vi "Abadines_Server5.vi"() -> ()   [LabVIEW 2013]
uses:
  <vilib>/NXT/Block Support/NXT_InputPort.ctl
  <vilib>/NXT/Block Support/NXT_MessageMailbox.ctl
  <vilib>/NXT/Block Support/NXT_OutputPort.ctl
  <vilib>/NXT/Subs/MotorOutput.ctl
  <vilib>/NXT/Dual Mode Library/BT/BlueTooth_Write_Num.vi
  <vilib>/NXT/NXTIO Xnodes/NXTIONodeSubVIs/NXTStopMotors.vi
  <vilib>/NXT/Dual Mode Library/Display/drawNumber.vi
  <vilib>/NXT/NXTIO Xnodes/AddressXNode/NXTIOAddress.xnode
  <vilib>/NXT/NXTIO Xnodes/NXTIOXNode/NXTIO.xnode
  <vilib>/NXT/Subs/LVHSConnector.ctl
  <vilib>/NXT/LegoClasses/BrickReference/BrickReference.lvclass
panel:
  out "Blue Line":i16
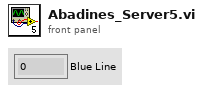
[diagram p1: front panel]
types:
  T1 = typedef "NXT_OutputPort.ctl" = u8
  T2 = typedef "NXT_InputPort.ctl" = u32
  T3 = typedef "LVHSConnector.ctl" = refnum<class "BrickReference.lvclass">
  T4 = typedef "NXT_MessageMailbox.ctl" = u8
  T5 = typedef "MotorOutput.ctl" = u8
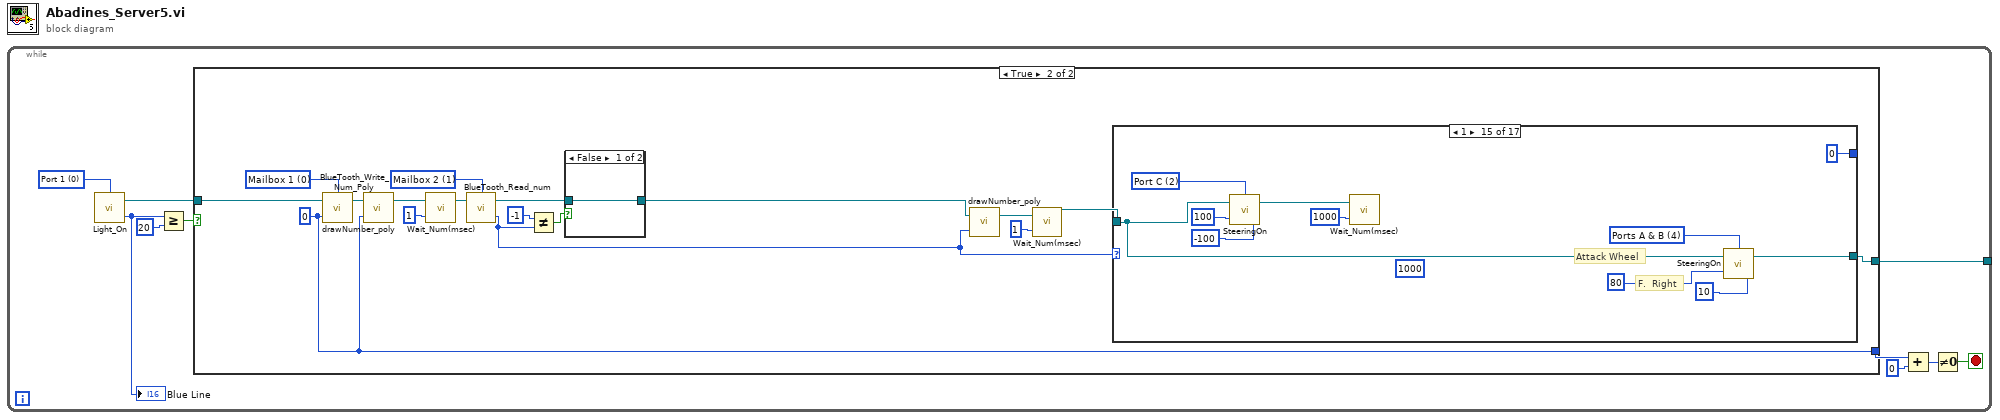
[diagram p0: block diagram]
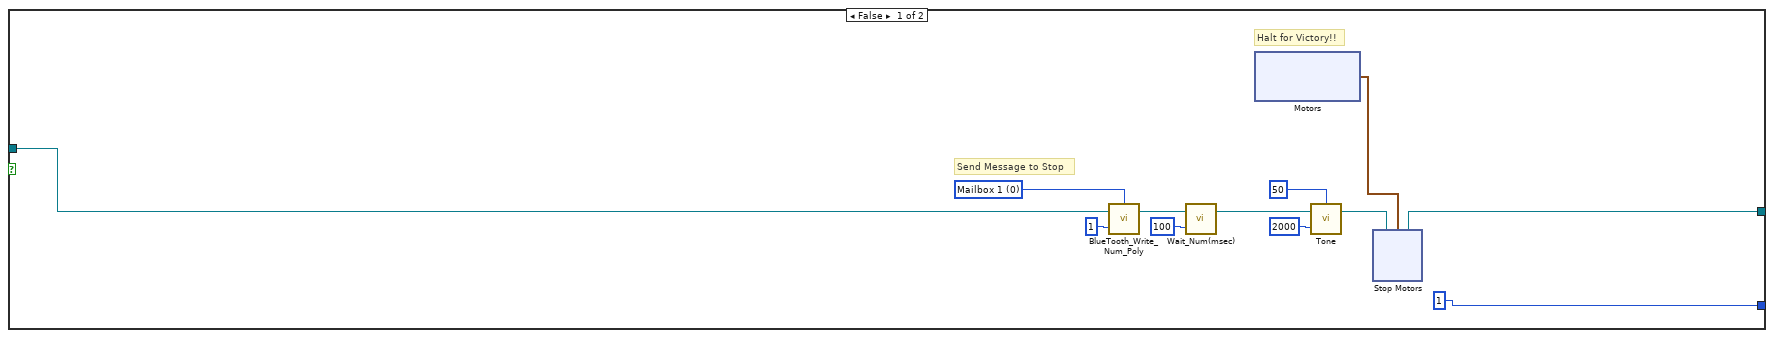
[diagram p2: hidden frame]
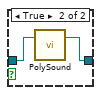
[diagram p3: hidden frame]
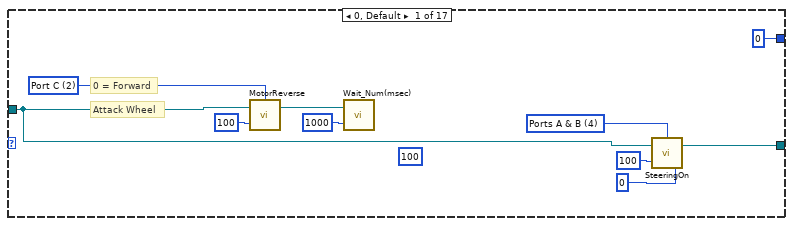
[diagram p4: hidden frame]
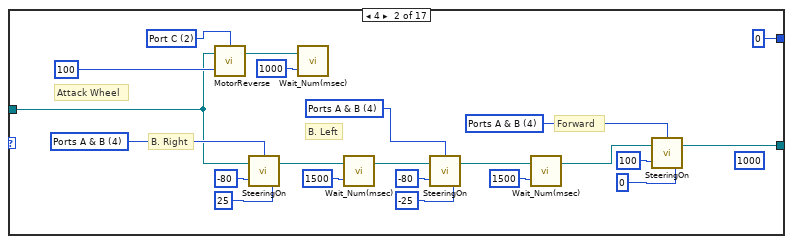
[diagram p5: hidden frame]
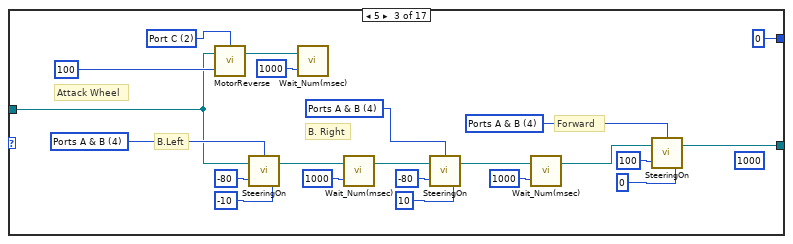
[diagram p6: hidden frame]
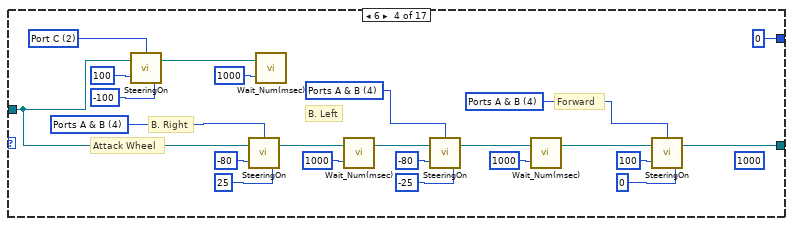
[diagram p7: hidden frame]
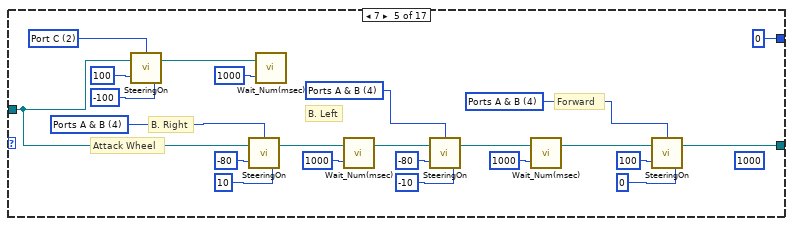
[diagram p8: hidden frame]
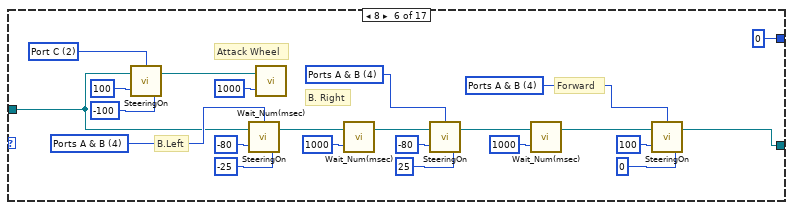
[diagram p9: hidden frame]
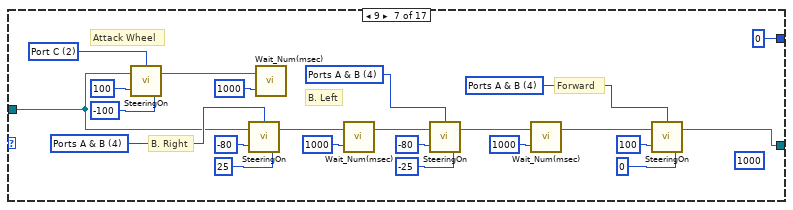
[diagram p10: hidden frame]
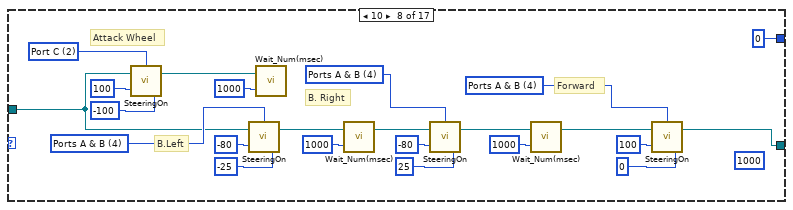
[diagram p11: hidden frame]
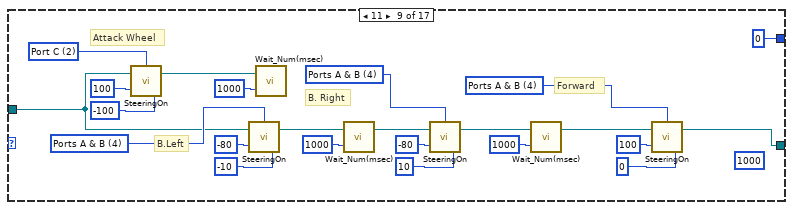
[diagram p12: hidden frame]
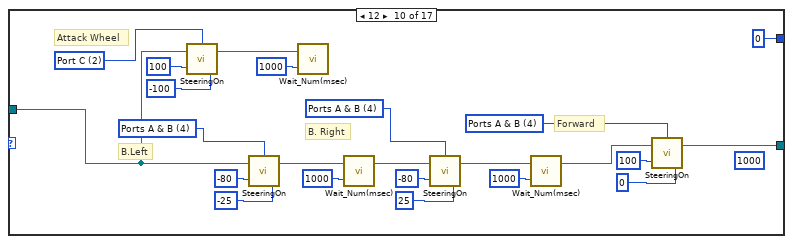
[diagram p13: hidden frame]
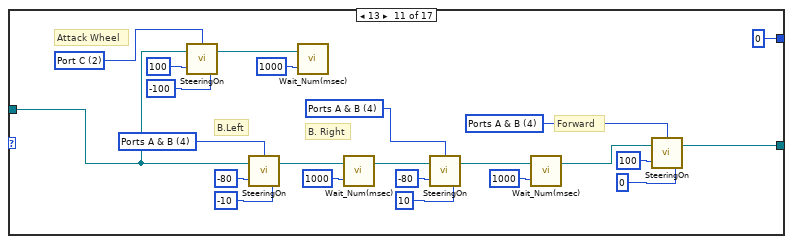
[diagram p14: hidden frame]
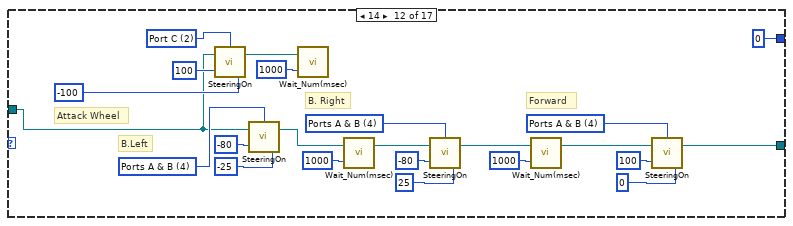
[diagram p15: hidden frame]
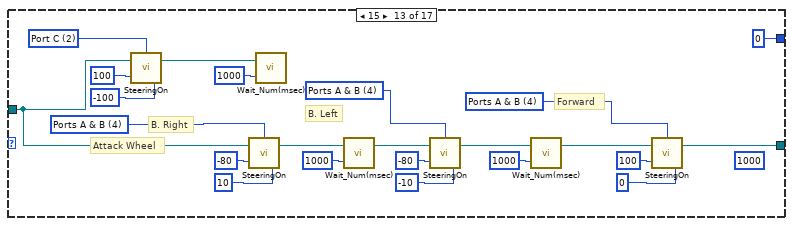
[diagram p16: hidden frame]
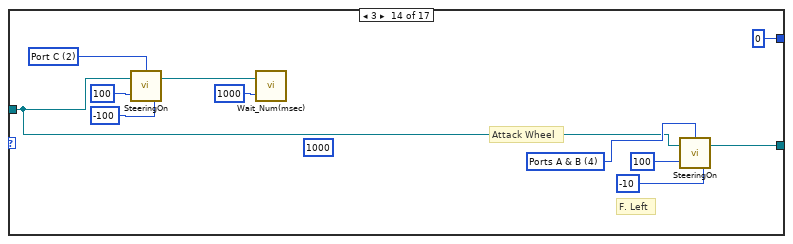
[diagram p17: hidden frame]
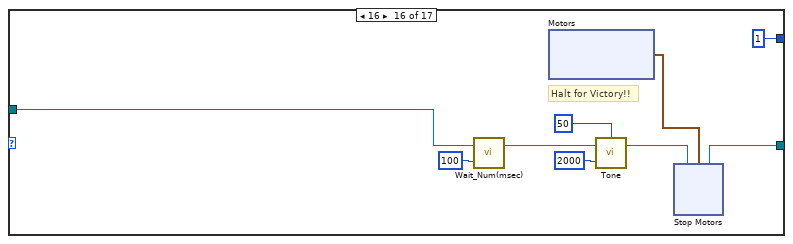
[diagram p18: hidden frame]
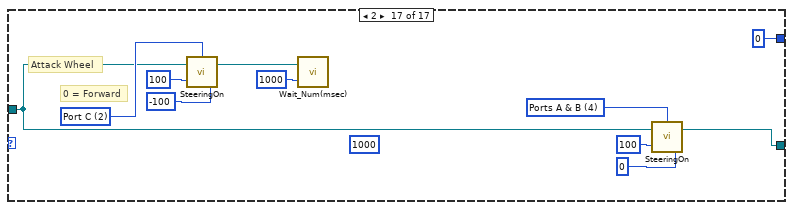
[diagram p19: hidden frame]
diagram:
  n1 = while {
    tunnel: [w6] -> _
    stop <- w2 stop-if-true
    w10 = T2 0 items=["Port 1", "Port 2", "Port 3", "Port 4"] ("Port (Port 3)")
    n2 = call <vilib>:"Light_On.vi"("Port (Port 3)"=w10) -> ("Scaled Value"=w9:i16, "NXT/EV3"=w1:T3)  [unwired: 2 in]
    "Blue Line" <- w9
    n3 = Greater Or Equal?(x=w9, y=i16 20) -> (x >= y?=w7:bool)
    n4 = case shown="True" w7 {
      tunnel: w1 -> [w20 w38]
      tunnel: [w14 w36] -> w6
      tunnel: [1 w35] -> w5
      frame False {
        w21 = T4 0 items=["Mailbox 1", "Mailbox 2", "Mailbox 3", "Mailbox 4", "Mailbox 5", "Mailbox 6", "Mailbox 7", "Mailbox 8", "Mailbox 9", "Mailbox 10"] ("Mailbox")
        # "Halt for Victory!!"
        # "Send Message to Stop"
        n5 = call-poly <vilib>:"BlueTooth_Write_Num_Poly.vi"("Message"=1, "NXT/EV3"=w20, "Mailbox"=w21) -> ("NXT/EV3"=w16:T3)  [unwired: 1 in]
        n6 = call <vilib>:"Wait_Num(msec).vi"("Time (100 msec)"=u32 100, "NXT/EV3"=w16) -> ("NXT/EV3"=w17:T3)  [unwired: 2 in]
        n7 = xnode "Motors"() -> ("Motor"=w13:cluster{"Port":T1, "Port":T1})
        n8 = call <vilib>:"Tone.vi"("Duration (500 ms)"=u16 2000, "NXT/EV3"=w17, "Tone (440 Hz)"=u16 50) -> ("NXT/EV3"=w15:T3)  [unwired: 1 in]
        n9 = xnode "Stop Motors"("Motors"=w13, "NXT/EV3"=w15) -> ("NXT/EV3"=w14:T3)
      }
      frame True {
        w45 = T4 1 items=["Mailbox 1", "Mailbox 2", "Mailbox 3", "Mailbox 4", "Mailbox 5", "Mailbox 6", "Mailbox 7", "Mailbox 8", "Mailbox 9", "Mailbox 10"] ("Mailbox")
        w35 = 0 ("Message")
        w39 = T4 0 items=["Mailbox 1", "Mailbox 2", "Mailbox 3", "Mailbox 4", "Mailbox 5", "Mailbox 6", "Mailbox 7", "Mailbox 8", "Mailbox 9", "Mailbox 10"] ("Mailbox")
        n10 = call-poly <vilib>:"BlueTooth_Write_Num_Poly.vi"("Message"=w35, "NXT/EV3"=w38, "Mailbox"=w39) -> ("NXT/EV3"=w32:T3)  [unwired: 1 in]
        n11 = call-poly <vilib>:"drawNumber_poly.vi"("number"=w35, "NXT/EV3"=w32) -> ("NXT/EV3"=w40:T3)  [unwired: 2 in]
        n12 = call <vilib>:"Wait_Num(msec).vi"("Time (100 msec)"=u32 1, "NXT/EV3"=w40) -> ("NXT/EV3"=w41:T3)  [unwired: 2 in]
        n13 = call <vilib>:"BlueTooth_Read_num.vi"("NXT/EV3"=w41, "Mailbox"=w45) -> ("Message"=w31:i32, "NXT/EV3"=w30:T3)  [unwired: 1 in]
        n14 = Not Equal?(x=-1, y=w31) -> (x != y?=w33:bool)
        n15 = case shown="False" w33 {
          tunnel: [w46 w48] -> w29
          tunnel: w30 -> [w46 w47]
          frame False {
          }
          frame True {
            n16 = call-poly <vilib>:"PolySound.vi"("NXT/EV3"=w47) -> ("NXT/EV3"=w48:T3)  [unwired: 3 in]
          }
        }
        n17 = call-poly <vilib>:"drawNumber_poly.vi"("number"=w31, "NXT/EV3"=w29) -> ("NXT/EV3"=w44:T3)  [unwired: 2 in]
        n18 = call <vilib>:"Wait_Num(msec).vi"("Time (100 msec)"=u32 1, "NXT/EV3"=w44) -> ("NXT/EV3"=w37:T3)  [unwired: 2 in]
        n19 = case shown="1" w31 {
          tunnel: [w56 w74 w87 w110 w133 w165 w179 w202 w225 w249 w271 w294 w318 w341 w352 w361 w378] -> w36
          tunnel: w37 -> [w49 w59 w81 w103 w126 w149 w172 w195 w218 w242 w265 w287 w310 w333 w344 w357 w371]
          tunnel: [0 ("Steering (100)") 0 ("Steering (100)") 0 ("Steering (100)") 0 ("Steering (100)") 0 ("Steering (100)") 0 ("Steering (100)") 0 ("Steering (100)") 0 ("Steering (100)") 0 ("Steering (100)") 0 ("Steering (100)") 0 ("Steering (100)") 0 ("Steering (100)") 0 ("Steering (100)") 0 ("Steering (100)") 0 ("Steering (100)") 1 ("Steering (100)") 0 ("Steering (100)")] -> _
          frame 0, Default {
            (unwired) u16 100 ("Duration (500 ms)")
            w54 = T5 2 items=["Port A"=0, "Port B"=1, "Port C"=2, "Ports A & B"=4, "Ports A & C"=5, "Ports B & C"=6, "All Ports"=3] ("Output Ports (A & B)")
            w55 = T5 4 items=["Port A"=0, "Port B"=1, "Port C"=2, "Ports A & B"=4, "Ports A & C"=5, "Ports B & C"=6, "All Ports"=3] ("Output Ports (A & B) 5")
            # "Attack Wheel"
            # "0 = Forward"
            n20 = call <vilib>:"MotorReverse.vi"("Power (75)"=100, "NXT/EV3"=w49, "Output Port (All Ports)"=w54) -> ("NXT/EV3"=w52:T3)  [unwired: 1 in]
            n21 = call <vilib>:"Wait_Num(msec).vi"("Time (100 msec)"=u32 1000, "NXT/EV3"=w52) -> ()  [unwired: 2 in, 1 out]
            n22 = call <vilib>:"SteeringOn.vi"("Power (75)"=100, "Steering (100)"=0, "NXT/EV3"=w49, "Output Ports (A & B)"=w55) -> ("NXT/EV3"=w56:T3)
          }
          frame 4 {
            (unwired) u16 1000 ("Duration (500 ms)")
            w64 = T5 2 items=["Port A"=0, "Port B"=1, "Port C"=2, "Ports A & B"=4, "Ports A & C"=5, "Ports B & C"=6, "All Ports"=3] ("Output Ports (A & B)")
            w71 = T5 4 items=["Port A"=0, "Port B"=1, "Port C"=2, "Ports A & B"=4, "Ports A & C"=5, "Ports B & C"=6, "All Ports"=3] ("Output Ports (A & B) 15")
            w72 = T5 4 items=["Port A"=0, "Port B"=1, "Port C"=2, "Ports A & B"=4, "Ports A & C"=5, "Ports B & C"=6, "All Ports"=3] ("Output Port (All Ports) 6")
            w73 = T5 4 items=["Port A"=0, "Port B"=1, "Port C"=2, "Ports A & B"=4, "Ports A & C"=5, "Ports B & C"=6, "All Ports"=3] ("Output Ports (A & B) 16")
            # "Attack Wheel"
            # "Forward"
            # "B. Left"
            # "B. Right"
            n23 = call <vilib>:"MotorReverse.vi"("Power (75)"=100, "NXT/EV3"=w59, "Output Port (All Ports)"=w64) -> ("NXT/EV3"=w62:T3)  [unwired: 1 in]
            n24 = call <vilib>:"SteeringOn.vi"("Power (75)"=-80, "Steering (100)"=25, "NXT/EV3"=w59, "Output Ports (A & B)"=w73) -> ("NXT/EV3"=w70:T3)
            n25 = call <vilib>:"Wait_Num(msec).vi"("Time (100 msec)"=u32 1000, "NXT/EV3"=w62) -> ()  [unwired: 2 in, 1 out]
            n26 = call <vilib>:"Wait_Num(msec).vi"("Time (100 msec)"=u32 1500, "NXT/EV3"=w70) -> ("NXT/EV3"=w69:T3)  [unwired: 2 in]
            n27 = call <vilib>:"SteeringOn.vi"("Power (75)"=-80, "Steering (100)"=-25, "NXT/EV3"=w69, "Output Ports (A & B)"=w72) -> ("NXT/EV3"=w68:T3)
            n28 = call <vilib>:"Wait_Num(msec).vi"("Time (100 msec)"=u32 1500, "NXT/EV3"=w68) -> ("NXT/EV3"=w67:T3)  [unwired: 2 in]
            n29 = call <vilib>:"SteeringOn.vi"("Power (75)"=100, "Steering (100)"=0, "NXT/EV3"=w67, "Output Ports (A & B)"=w71) -> ("NXT/EV3"=w74:T3)
          }
          frame 5 {
            (unwired) u16 1000 ("Duration (500 ms)")
            w86 = T5 2 items=["Port A"=0, "Port B"=1, "Port C"=2, "Ports A & B"=4, "Ports A & C"=5, "Ports B & C"=6, "All Ports"=3] ("Output Ports (A & B)")
            w94 = T5 4 items=["Port A"=0, "Port B"=1, "Port C"=2, "Ports A & B"=4, "Ports A & C"=5, "Ports B & C"=6, "All Ports"=3] ("Output Ports (A & B) 21")
            w95 = T5 4 items=["Port A"=0, "Port B"=1, "Port C"=2, "Ports A & B"=4, "Ports A & C"=5, "Ports B & C"=6, "All Ports"=3] ("Output Port (All Ports) 9")
            w96 = T5 4 items=["Port A"=0, "Port B"=1, "Port C"=2, "Ports A & B"=4, "Ports A & C"=5, "Ports B & C"=6, "All Ports"=3] ("Output Ports (A & B) 22")
            # "Attack Wheel"
            # "Forward"
            # "B. Right"
            # "B.Left"
            n30 = call <vilib>:"MotorReverse.vi"("Power (75)"=100, "NXT/EV3"=w81, "Output Port (All Ports)"=w86) -> ("NXT/EV3"=w84:T3)  [unwired: 1 in]
            n31 = call <vilib>:"SteeringOn.vi"("Power (75)"=-80, "Steering (100)"=-10, "NXT/EV3"=w81, "Output Ports (A & B)"=w96) -> ("NXT/EV3"=w92:T3)
            n32 = call <vilib>:"Wait_Num(msec).vi"("Time (100 msec)"=u32 1000, "NXT/EV3"=w84) -> ()  [unwired: 2 in, 1 out]
            n33 = call <vilib>:"Wait_Num(msec).vi"("Time (100 msec)"=u32 1000, "NXT/EV3"=w92) -> ("NXT/EV3"=w91:T3)  [unwired: 2 in]
            n34 = call <vilib>:"SteeringOn.vi"("Power (75)"=-80, "Steering (100)"=10, "NXT/EV3"=w91, "Output Ports (A & B)"=w95) -> ("NXT/EV3"=w89:T3)
            n35 = call <vilib>:"Wait_Num(msec).vi"("Time (100 msec)"=u32 1000, "NXT/EV3"=w89) -> ("NXT/EV3"=w88:T3)  [unwired: 2 in]
            n36 = call <vilib>:"SteeringOn.vi"("Power (75)"=100, "Steering (100)"=0, "NXT/EV3"=w88, "Output Ports (A & B)"=w94) -> ("NXT/EV3"=w87:T3)
          }
          frame 6 {
            (unwired) u16 1000 ("Duration (500 ms)")
            w109 = T5 2 items=["Port A"=0, "Port B"=1, "Port C"=2, "Ports A & B"=4, "Ports A & C"=5, "Ports B & C"=6, "All Ports"=3] ("Output Ports (A & B)")
            w119 = T5 4 items=["Port A"=0, "Port B"=1, "Port C"=2, "Ports A & B"=4, "Ports A & C"=5, "Ports B & C"=6, "All Ports"=3] ("Output Ports (A & B) 15")
            w118 = T5 4 items=["Port A"=0, "Port B"=1, "Port C"=2, "Ports A & B"=4, "Ports A & C"=5, "Ports B & C"=6, "All Ports"=3] ("Output Port (All Ports) 6")
            w117 = T5 4 items=["Port A"=0, "Port B"=1, "Port C"=2, "Ports A & B"=4, "Ports A & C"=5, "Ports B & C"=6, "All Ports"=3] ("Output Ports (A & B) 16")
            # "Attack Wheel"
            # "Forward"
            # "B. Left"
            # "B. Right"
            n37 = call <vilib>:"SteeringOn.vi"("Power (75)"=100, "Steering (100)"=-100, "NXT/EV3"=w103, "Output Ports (A & B)"=w109) -> ("NXT/EV3"=w106:T3)
            n38 = call <vilib>:"SteeringOn.vi"("Power (75)"=-80, "Steering (100)"=25, "NXT/EV3"=w103, "Output Ports (A & B)"=w117) -> ("NXT/EV3"=w120:T3)
            n39 = call <vilib>:"Wait_Num(msec).vi"("Time (100 msec)"=u32 1000, "NXT/EV3"=w106) -> ()  [unwired: 2 in, 1 out]
            n40 = call <vilib>:"Wait_Num(msec).vi"("Time (100 msec)"=u32 1000, "NXT/EV3"=w120) -> ("NXT/EV3"=w121:T3)  [unwired: 2 in]
            n41 = call <vilib>:"SteeringOn.vi"("Power (75)"=-80, "Steering (100)"=-25, "NXT/EV3"=w121, "Output Ports (A & B)"=w118) -> ("NXT/EV3"=w122:T3)
            n42 = call <vilib>:"Wait_Num(msec).vi"("Time (100 msec)"=u32 1000, "NXT/EV3"=w122) -> ("NXT/EV3"=w123:T3)  [unwired: 2 in]
            n43 = call <vilib>:"SteeringOn.vi"("Power (75)"=100, "Steering (100)"=0, "NXT/EV3"=w123, "Output Ports (A & B)"=w119) -> ("NXT/EV3"=w110:T3)
          }
          frame 7 {
            (unwired) u16 1000 ("Duration (500 ms)")
            w132 = T5 2 items=["Port A"=0, "Port B"=1, "Port C"=2, "Ports A & B"=4, "Ports A & C"=5, "Ports B & C"=6, "All Ports"=3] ("Output Ports (A & B)")
            w142 = T5 4 items=["Port A"=0, "Port B"=1, "Port C"=2, "Ports A & B"=4, "Ports A & C"=5, "Ports B & C"=6, "All Ports"=3] ("Output Ports (A & B) 15")
            w141 = T5 4 items=["Port A"=0, "Port B"=1, "Port C"=2, "Ports A & B"=4, "Ports A & C"=5, "Ports B & C"=6, "All Ports"=3] ("Output Port (All Ports) 6")
            w140 = T5 4 items=["Port A"=0, "Port B"=1, "Port C"=2, "Ports A & B"=4, "Ports A & C"=5, "Ports B & C"=6, "All Ports"=3] ("Output Ports (A & B) 16")
            # "Attack Wheel"
            # "Forward"
            # "B. Left"
            # "B. Right"
            n44 = call <vilib>:"SteeringOn.vi"("Power (75)"=100, "Steering (100)"=-100, "NXT/EV3"=w126, "Output Ports (A & B)"=w132) -> ("NXT/EV3"=w129:T3)
            n45 = call <vilib>:"SteeringOn.vi"("Power (75)"=-80, "Steering (100)"=10, "NXT/EV3"=w126, "Output Ports (A & B)"=w140) -> ("NXT/EV3"=w143:T3)
            n46 = call <vilib>:"Wait_Num(msec).vi"("Time (100 msec)"=u32 1000, "NXT/EV3"=w129) -> ()  [unwired: 2 in, 1 out]
            n47 = call <vilib>:"Wait_Num(msec).vi"("Time (100 msec)"=u32 1000, "NXT/EV3"=w143) -> ("NXT/EV3"=w144:T3)  [unwired: 2 in]
            n48 = call <vilib>:"SteeringOn.vi"("Power (75)"=-80, "Steering (100)"=-10, "NXT/EV3"=w144, "Output Ports (A & B)"=w141) -> ("NXT/EV3"=w145:T3)
            n49 = call <vilib>:"Wait_Num(msec).vi"("Time (100 msec)"=u32 1000, "NXT/EV3"=w145) -> ("NXT/EV3"=w146:T3)  [unwired: 2 in]
            n50 = call <vilib>:"SteeringOn.vi"("Power (75)"=100, "Steering (100)"=0, "NXT/EV3"=w146, "Output Ports (A & B)"=w142) -> ("NXT/EV3"=w133:T3)
          }
          frame 8 {
            w155 = T5 2 items=["Port A"=0, "Port B"=1, "Port C"=2, "Ports A & B"=4, "Ports A & C"=5, "Ports B & C"=6, "All Ports"=3] ("Output Ports (A & B)")
            w162 = T5 4 items=["Port A"=0, "Port B"=1, "Port C"=2, "Ports A & B"=4, "Ports A & C"=5, "Ports B & C"=6, "All Ports"=3] ("Output Ports (A & B) 21")
            w163 = T5 4 items=["Port A"=0, "Port B"=1, "Port C"=2, "Ports A & B"=4, "Ports A & C"=5, "Ports B & C"=6, "All Ports"=3] ("Output Port (All Ports) 9")
            w164 = T5 4 items=["Port A"=0, "Port B"=1, "Port C"=2, "Ports A & B"=4, "Ports A & C"=5, "Ports B & C"=6, "All Ports"=3] ("Output Ports (A & B) 22")
            # "Attack Wheel"
            # "Forward"
            # "B. Right"
            # "B.Left"
            n51 = call <vilib>:"SteeringOn.vi"("Power (75)"=100, "Steering (100)"=-100, "NXT/EV3"=w149, "Output Ports (A & B)"=w155) -> ("NXT/EV3"=w152:T3)
            n52 = call <vilib>:"SteeringOn.vi"("Power (75)"=-80, "Steering (100)"=-25, "NXT/EV3"=w149, "Output Ports (A & B)"=w164) -> ("NXT/EV3"=w160:T3)
            n53 = call <vilib>:"Wait_Num(msec).vi"("Time (100 msec)"=u32 1000, "NXT/EV3"=w152) -> ()  [unwired: 2 in, 1 out]
            n54 = call <vilib>:"Wait_Num(msec).vi"("Time (100 msec)"=u32 1000, "NXT/EV3"=w160) -> ("NXT/EV3"=w159:T3)  [unwired: 2 in]
            n55 = call <vilib>:"SteeringOn.vi"("Power (75)"=-80, "Steering (100)"=25, "NXT/EV3"=w159, "Output Ports (A & B)"=w163) -> ("NXT/EV3"=w157:T3)
            n56 = call <vilib>:"Wait_Num(msec).vi"("Time (100 msec)"=u32 1000, "NXT/EV3"=w157) -> ("NXT/EV3"=w156:T3)  [unwired: 2 in]
            n57 = call <vilib>:"SteeringOn.vi"("Power (75)"=100, "Steering (100)"=0, "NXT/EV3"=w156, "Output Ports (A & B)"=w162) -> ("NXT/EV3"=w165:T3)
          }
          frame 9 {
            (unwired) u16 1000 ("Duration (500 ms)")
            w178 = T5 2 items=["Port A"=0, "Port B"=1, "Port C"=2, "Ports A & B"=4, "Ports A & C"=5, "Ports B & C"=6, "All Ports"=3] ("Output Ports (A & B)")
            w186 = T5 4 items=["Port A"=0, "Port B"=1, "Port C"=2, "Ports A & B"=4, "Ports A & C"=5, "Ports B & C"=6, "All Ports"=3] ("Output Ports (A & B) 15")
            w187 = T5 4 items=["Port A"=0, "Port B"=1, "Port C"=2, "Ports A & B"=4, "Ports A & C"=5, "Ports B & C"=6, "All Ports"=3] ("Output Port (All Ports) 6")
            w188 = T5 4 items=["Port A"=0, "Port B"=1, "Port C"=2, "Ports A & B"=4, "Ports A & C"=5, "Ports B & C"=6, "All Ports"=3] ("Output Ports (A & B) 16")
            # "Attack Wheel"
            # "Forward"
            # "B. Left"
            # "B. Right"
            n58 = call <vilib>:"SteeringOn.vi"("Power (75)"=100, "Steering (100)"=-100, "NXT/EV3"=w172, "Output Ports (A & B)"=w178) -> ("NXT/EV3"=w175:T3)
            n59 = call <vilib>:"SteeringOn.vi"("Power (75)"=-80, "Steering (100)"=25, "NXT/EV3"=w172, "Output Ports (A & B)"=w188) -> ("NXT/EV3"=w185:T3)
            n60 = call <vilib>:"Wait_Num(msec).vi"("Time (100 msec)"=u32 1000, "NXT/EV3"=w175) -> ()  [unwired: 2 in, 1 out]
            n61 = call <vilib>:"Wait_Num(msec).vi"("Time (100 msec)"=u32 1000, "NXT/EV3"=w185) -> ("NXT/EV3"=w184:T3)  [unwired: 2 in]
            n62 = call <vilib>:"SteeringOn.vi"("Power (75)"=-80, "Steering (100)"=-25, "NXT/EV3"=w184, "Output Ports (A & B)"=w187) -> ("NXT/EV3"=w183:T3)
            n63 = call <vilib>:"Wait_Num(msec).vi"("Time (100 msec)"=u32 1000, "NXT/EV3"=w183) -> ("NXT/EV3"=w182:T3)  [unwired: 2 in]
            n64 = call <vilib>:"SteeringOn.vi"("Power (75)"=100, "Steering (100)"=0, "NXT/EV3"=w182, "Output Ports (A & B)"=w186) -> ("NXT/EV3"=w179:T3)
          }
          frame 10 {
            (unwired) u16 1000 ("Duration (500 ms)")
            w201 = T5 2 items=["Port A"=0, "Port B"=1, "Port C"=2, "Ports A & B"=4, "Ports A & C"=5, "Ports B & C"=6, "All Ports"=3] ("Output Ports (A & B)")
            w211 = T5 4 items=["Port A"=0, "Port B"=1, "Port C"=2, "Ports A & B"=4, "Ports A & C"=5, "Ports B & C"=6, "All Ports"=3] ("Output Ports (A & B) 21")
            w210 = T5 4 items=["Port A"=0, "Port B"=1, "Port C"=2, "Ports A & B"=4, "Ports A & C"=5, "Ports B & C"=6, "All Ports"=3] ("Output Port (All Ports) 9")
            w209 = T5 4 items=["Port A"=0, "Port B"=1, "Port C"=2, "Ports A & B"=4, "Ports A & C"=5, "Ports B & C"=6, "All Ports"=3] ("Output Ports (A & B) 22")
            # "Attack Wheel"
            # "Forward"
            # "B. Right"
            # "B.Left"
            n65 = call <vilib>:"SteeringOn.vi"("Power (75)"=100, "Steering (100)"=-100, "NXT/EV3"=w195, "Output Ports (A & B)"=w201) -> ("NXT/EV3"=w198:T3)
            n66 = call <vilib>:"SteeringOn.vi"("Power (75)"=-80, "Steering (100)"=-25, "NXT/EV3"=w195, "Output Ports (A & B)"=w209) -> ("NXT/EV3"=w213:T3)
            n67 = call <vilib>:"Wait_Num(msec).vi"("Time (100 msec)"=u32 1000, "NXT/EV3"=w198) -> ()  [unwired: 2 in, 1 out]
            n68 = call <vilib>:"Wait_Num(msec).vi"("Time (100 msec)"=u32 1000, "NXT/EV3"=w213) -> ("NXT/EV3"=w214:T3)  [unwired: 2 in]
            n69 = call <vilib>:"SteeringOn.vi"("Power (75)"=-80, "Steering (100)"=25, "NXT/EV3"=w214, "Output Ports (A & B)"=w210) -> ("NXT/EV3"=w216:T3)
            n70 = call <vilib>:"Wait_Num(msec).vi"("Time (100 msec)"=u32 1000, "NXT/EV3"=w216) -> ("NXT/EV3"=w217:T3)  [unwired: 2 in]
            n71 = call <vilib>:"SteeringOn.vi"("Power (75)"=100, "Steering (100)"=0, "NXT/EV3"=w217, "Output Ports (A & B)"=w211) -> ("NXT/EV3"=w202:T3)
          }
          frame 11 {
            (unwired) u16 1000 ("Duration (500 ms)")
            w224 = T5 2 items=["Port A"=0, "Port B"=1, "Port C"=2, "Ports A & B"=4, "Ports A & C"=5, "Ports B & C"=6, "All Ports"=3] ("Output Ports (A & B)")
            w234 = T5 4 items=["Port A"=0, "Port B"=1, "Port C"=2, "Ports A & B"=4, "Ports A & C"=5, "Ports B & C"=6, "All Ports"=3] ("Output Ports (A & B) 21")
            w233 = T5 4 items=["Port A"=0, "Port B"=1, "Port C"=2, "Ports A & B"=4, "Ports A & C"=5, "Ports B & C"=6, "All Ports"=3] ("Output Port (All Ports) 9")
            w232 = T5 4 items=["Port A"=0, "Port B"=1, "Port C"=2, "Ports A & B"=4, "Ports A & C"=5, "Ports B & C"=6, "All Ports"=3] ("Output Ports (A & B) 22")
            # "Attack Wheel"
            # "Forward"
            # "B. Right"
            # "B.Left"
            n72 = call <vilib>:"SteeringOn.vi"("Power (75)"=100, "Steering (100)"=-100, "NXT/EV3"=w218, "Output Ports (A & B)"=w224) -> ("NXT/EV3"=w221:T3)
            n73 = call <vilib>:"SteeringOn.vi"("Power (75)"=-80, "Steering (100)"=-10, "NXT/EV3"=w218, "Output Ports (A & B)"=w232) -> ("NXT/EV3"=w236:T3)
            n74 = call <vilib>:"Wait_Num(msec).vi"("Time (100 msec)"=u32 1000, "NXT/EV3"=w221) -> ()  [unwired: 2 in, 1 out]
            n75 = call <vilib>:"Wait_Num(msec).vi"("Time (100 msec)"=u32 1000, "NXT/EV3"=w236) -> ("NXT/EV3"=w237:T3)  [unwired: 2 in]
            n76 = call <vilib>:"SteeringOn.vi"("Power (75)"=-80, "Steering (100)"=10, "NXT/EV3"=w237, "Output Ports (A & B)"=w233) -> ("NXT/EV3"=w239:T3)
            n77 = call <vilib>:"Wait_Num(msec).vi"("Time (100 msec)"=u32 1000, "NXT/EV3"=w239) -> ("NXT/EV3"=w240:T3)  [unwired: 2 in]
            n78 = call <vilib>:"SteeringOn.vi"("Power (75)"=100, "Steering (100)"=0, "NXT/EV3"=w240, "Output Ports (A & B)"=w234) -> ("NXT/EV3"=w225:T3)
          }
          frame 12 {
            (unwired) u16 1000 ("Duration (500 ms)")
            w248 = T5 2 items=["Port A"=0, "Port B"=1, "Port C"=2, "Ports A & B"=4, "Ports A & C"=5, "Ports B & C"=6, "All Ports"=3] ("Output Ports (A & B)")
            w257 = T5 4 items=["Port A"=0, "Port B"=1, "Port C"=2, "Ports A & B"=4, "Ports A & C"=5, "Ports B & C"=6, "All Ports"=3] ("Output Ports (A & B) 21")
            w256 = T5 4 items=["Port A"=0, "Port B"=1, "Port C"=2, "Ports A & B"=4, "Ports A & C"=5, "Ports B & C"=6, "All Ports"=3] ("Output Port (All Ports) 9")
            w241 = T5 4 items=["Port A"=0, "Port B"=1, "Port C"=2, "Ports A & B"=4, "Ports A & C"=5, "Ports B & C"=6, "All Ports"=3] ("Output Ports (A & B) 22")
            # "Attack Wheel"
            # "Forward"
            # "B. Right"
            # "B.Left"
            n79 = call <vilib>:"SteeringOn.vi"("Power (75)"=100, "Steering (100)"=-100, "NXT/EV3"=w242, "Output Ports (A & B)"=w248) -> ("NXT/EV3"=w245:T3)
            n80 = call <vilib>:"SteeringOn.vi"("Power (75)"=-80, "Steering (100)"=-25, "NXT/EV3"=w242, "Output Ports (A & B)"=w241) -> ("NXT/EV3"=w259:T3)
            n81 = call <vilib>:"Wait_Num(msec).vi"("Time (100 msec)"=u32 1000, "NXT/EV3"=w245) -> ()  [unwired: 2 in, 1 out]
            n82 = call <vilib>:"Wait_Num(msec).vi"("Time (100 msec)"=u32 1000, "NXT/EV3"=w259) -> ("NXT/EV3"=w260:T3)  [unwired: 2 in]
            n83 = call <vilib>:"SteeringOn.vi"("Power (75)"=-80, "Steering (100)"=25, "NXT/EV3"=w260, "Output Ports (A & B)"=w256) -> ("NXT/EV3"=w262:T3)
            n84 = call <vilib>:"Wait_Num(msec).vi"("Time (100 msec)"=u32 1000, "NXT/EV3"=w262) -> ("NXT/EV3"=w263:T3)  [unwired: 2 in]
            n85 = call <vilib>:"SteeringOn.vi"("Power (75)"=100, "Steering (100)"=0, "NXT/EV3"=w263, "Output Ports (A & B)"=w257) -> ("NXT/EV3"=w249:T3)
          }
          frame 13 {
            w270 = T5 2 items=["Port A"=0, "Port B"=1, "Port C"=2, "Ports A & B"=4, "Ports A & C"=5, "Ports B & C"=6, "All Ports"=3] ("Output Ports (A & B)")
            w278 = T5 4 items=["Port A"=0, "Port B"=1, "Port C"=2, "Ports A & B"=4, "Ports A & C"=5, "Ports B & C"=6, "All Ports"=3] ("Output Ports (A & B) 21")
            w279 = T5 4 items=["Port A"=0, "Port B"=1, "Port C"=2, "Ports A & B"=4, "Ports A & C"=5, "Ports B & C"=6, "All Ports"=3] ("Output Port (All Ports) 9")
            w280 = T5 4 items=["Port A"=0, "Port B"=1, "Port C"=2, "Ports A & B"=4, "Ports A & C"=5, "Ports B & C"=6, "All Ports"=3] ("Output Ports (A & B) 22")
            # "Attack Wheel"
            # "Forward"
            # "B. Right"
            # "B.Left"
            n86 = call <vilib>:"SteeringOn.vi"("Power (75)"=100, "Steering (100)"=-100, "NXT/EV3"=w265, "Output Ports (A & B)"=w270) -> ("NXT/EV3"=w267:T3)
            n87 = call <vilib>:"SteeringOn.vi"("Power (75)"=-80, "Steering (100)"=-10, "NXT/EV3"=w265, "Output Ports (A & B)"=w280) -> ("NXT/EV3"=w276:T3)
            n88 = call <vilib>:"Wait_Num(msec).vi"("Time (100 msec)"=u32 1000, "NXT/EV3"=w267) -> ()  [unwired: 2 in, 1 out]
            n89 = call <vilib>:"Wait_Num(msec).vi"("Time (100 msec)"=u32 1000, "NXT/EV3"=w276) -> ("NXT/EV3"=w275:T3)  [unwired: 2 in]
            n90 = call <vilib>:"SteeringOn.vi"("Power (75)"=-80, "Steering (100)"=10, "NXT/EV3"=w275, "Output Ports (A & B)"=w279) -> ("NXT/EV3"=w273:T3)
            n91 = call <vilib>:"Wait_Num(msec).vi"("Time (100 msec)"=u32 1000, "NXT/EV3"=w273) -> ("NXT/EV3"=w272:T3)  [unwired: 2 in]
            n92 = call <vilib>:"SteeringOn.vi"("Power (75)"=100, "Steering (100)"=0, "NXT/EV3"=w272, "Output Ports (A & B)"=w278) -> ("NXT/EV3"=w271:T3)
          }
          frame 14 {
            w293 = T5 2 items=["Port A"=0, "Port B"=1, "Port C"=2, "Ports A & B"=4, "Ports A & C"=5, "Ports B & C"=6, "All Ports"=3] ("Output Ports (A & B)")
            w303 = T5 4 items=["Port A"=0, "Port B"=1, "Port C"=2, "Ports A & B"=4, "Ports A & C"=5, "Ports B & C"=6, "All Ports"=3] ("Output Ports (A & B) 21")
            w302 = T5 4 items=["Port A"=0, "Port B"=1, "Port C"=2, "Ports A & B"=4, "Ports A & C"=5, "Ports B & C"=6, "All Ports"=3] ("Output Port (All Ports) 9")
            w301 = T5 4 items=["Port A"=0, "Port B"=1, "Port C"=2, "Ports A & B"=4, "Ports A & C"=5, "Ports B & C"=6, "All Ports"=3] ("Output Ports (A & B) 22")
            # "Attack Wheel"
            # "Forward"
            # "B. Right"
            # "B.Left"
            n93 = call <vilib>:"SteeringOn.vi"("Power (75)"=100, "Steering (100)"=-100, "NXT/EV3"=w287, "Output Ports (A & B)"=w293) -> ("NXT/EV3"=w290:T3)
            n94 = call <vilib>:"SteeringOn.vi"("Power (75)"=-80, "Steering (100)"=-25, "NXT/EV3"=w287, "Output Ports (A & B)"=w301) -> ("NXT/EV3"=w305:T3)
            n95 = call <vilib>:"Wait_Num(msec).vi"("Time (100 msec)"=u32 1000, "NXT/EV3"=w290) -> ()  [unwired: 2 in, 1 out]
            n96 = call <vilib>:"Wait_Num(msec).vi"("Time (100 msec)"=u32 1000, "NXT/EV3"=w305) -> ("NXT/EV3"=w306:T3)  [unwired: 2 in]
            n97 = call <vilib>:"SteeringOn.vi"("Power (75)"=-80, "Steering (100)"=25, "NXT/EV3"=w306, "Output Ports (A & B)"=w302) -> ("NXT/EV3"=w308:T3)
            n98 = call <vilib>:"Wait_Num(msec).vi"("Time (100 msec)"=u32 1000, "NXT/EV3"=w308) -> ("NXT/EV3"=w309:T3)  [unwired: 2 in]
            n99 = call <vilib>:"SteeringOn.vi"("Power (75)"=100, "Steering (100)"=0, "NXT/EV3"=w309, "Output Ports (A & B)"=w303) -> ("NXT/EV3"=w294:T3)
          }
          frame 15 {
            (unwired) u16 1000 ("Duration (500 ms)")
            w316 = T5 2 items=["Port A"=0, "Port B"=1, "Port C"=2, "Ports A & B"=4, "Ports A & C"=5, "Ports B & C"=6, "All Ports"=3] ("Output Ports (A & B)")
            w325 = T5 4 items=["Port A"=0, "Port B"=1, "Port C"=2, "Ports A & B"=4, "Ports A & C"=5, "Ports B & C"=6, "All Ports"=3] ("Output Ports (A & B) 15")
            w326 = T5 4 items=["Port A"=0, "Port B"=1, "Port C"=2, "Ports A & B"=4, "Ports A & C"=5, "Ports B & C"=6, "All Ports"=3] ("Output Port (All Ports) 6")
            w317 = T5 4 items=["Port A"=0, "Port B"=1, "Port C"=2, "Ports A & B"=4, "Ports A & C"=5, "Ports B & C"=6, "All Ports"=3] ("Output Ports (A & B) 16")
            # "Attack Wheel"
            # "Forward"
            # "B. Left"
            # "B. Right"
            n100 = call <vilib>:"SteeringOn.vi"("Power (75)"=100, "Steering (100)"=-100, "NXT/EV3"=w310, "Output Ports (A & B)"=w316) -> ("NXT/EV3"=w313:T3)
            n101 = call <vilib>:"SteeringOn.vi"("Power (75)"=-80, "Steering (100)"=10, "NXT/EV3"=w310, "Output Ports (A & B)"=w317) -> ("NXT/EV3"=w324:T3)
            n102 = call <vilib>:"Wait_Num(msec).vi"("Time (100 msec)"=u32 1000, "NXT/EV3"=w313) -> ()  [unwired: 2 in, 1 out]
            n103 = call <vilib>:"Wait_Num(msec).vi"("Time (100 msec)"=u32 1000, "NXT/EV3"=w324) -> ("NXT/EV3"=w323:T3)  [unwired: 2 in]
            n104 = call <vilib>:"SteeringOn.vi"("Power (75)"=-80, "Steering (100)"=-10, "NXT/EV3"=w323, "Output Ports (A & B)"=w326) -> ("NXT/EV3"=w322:T3)
            n105 = call <vilib>:"Wait_Num(msec).vi"("Time (100 msec)"=u32 1000, "NXT/EV3"=w322) -> ("NXT/EV3"=w321:T3)  [unwired: 2 in]
            n106 = call <vilib>:"SteeringOn.vi"("Power (75)"=100, "Steering (100)"=0, "NXT/EV3"=w321, "Output Ports (A & B)"=w325) -> ("NXT/EV3"=w318:T3)
          }
          frame 3 {
            (unwired) u16 1000 ("Duration (500 ms)")
            w339 = T5 2 items=["Port A"=0, "Port B"=1, "Port C"=2, "Ports A & B"=4, "Ports A & C"=5, "Ports B & C"=6, "All Ports"=3] ("Output Ports (A & B)")
            w340 = T5 4 items=["Port A"=0, "Port B"=1, "Port C"=2, "Ports A & B"=4, "Ports A & C"=5, "Ports B & C"=6, "All Ports"=3] ("Output Port (All Ports) 3")
            # "Attack Wheel"
            # "F. Left"
            n107 = call <vilib>:"SteeringOn.vi"("Power (75)"=100, "Steering (100)"=-100, "NXT/EV3"=w333, "Output Ports (A & B)"=w339) -> ("NXT/EV3"=w336:T3)
            n108 = call <vilib>:"Wait_Num(msec).vi"("Time (100 msec)"=u32 1000, "NXT/EV3"=w336) -> ()  [unwired: 2 in, 1 out]
            n109 = call <vilib>:"SteeringOn.vi"("Power (75)"=100, "Steering (100)"=-10, "NXT/EV3"=w333, "Output Ports (A & B)"=w340) -> ("NXT/EV3"=w341:T3)
          }
          frame 1 {
            (unwired) u16 1000 ("Duration (500 ms)")
            w350 = T5 2 items=["Port A"=0, "Port B"=1, "Port C"=2, "Ports A & B"=4, "Ports A & C"=5, "Ports B & C"=6, "All Ports"=3] ("Output Ports (A & B)")
            w351 = T5 4 items=["Port A"=0, "Port B"=1, "Port C"=2, "Ports A & B"=4, "Ports A & C"=5, "Ports B & C"=6, "All Ports"=3] ("Output Ports (A & B) 12")
            # "Attack Wheel"
            # "F.  Right"
            n110 = call <vilib>:"SteeringOn.vi"("Power (75)"=100, "Steering (100)"=-100, "NXT/EV3"=w344, "Output Ports (A & B)"=w350) -> ("NXT/EV3"=w347:T3)
            n111 = call <vilib>:"Wait_Num(msec).vi"("Time (100 msec)"=u32 1000, "NXT/EV3"=w347) -> ()  [unwired: 2 in, 1 out]
            n112 = call <vilib>:"SteeringOn.vi"("Power (75)"=80, "Steering (100)"=10, "NXT/EV3"=w344, "Output Ports (A & B)"=w351) -> ("NXT/EV3"=w352:T3)
          }
          frame 16 {
            # "Halt for Victory!!"
            n113 = call <vilib>:"Wait_Num(msec).vi"("Time (100 msec)"=u32 100, "NXT/EV3"=w357) -> ("NXT/EV3"=w360:T3)  [unwired: 2 in]
            n114 = xnode "Motors"() -> ("Motor"=w363:cluster{"Port":T1, "Port":T1})
            n115 = call <vilib>:"Tone.vi"("Duration (500 ms)"=u16 2000, "NXT/EV3"=w360, "Tone (440 Hz)"=u16 50) -> ("NXT/EV3"=w359:T3)  [unwired: 1 in]
            n116 = xnode "Stop Motors"("Motors"=w363, "NXT/EV3"=w359) -> ("NXT/EV3"=w361:T3)
          }
          frame 2 {
            (unwired) u16 1000 ("Duration (500 ms)")
            w376 = T5 2 items=["Port A"=0, "Port B"=1, "Port C"=2, "Ports A & B"=4, "Ports A & C"=5, "Ports B & C"=6, "All Ports"=3] ("Output Ports (A & B)")
            w377 = T5 4 items=["Port A"=0, "Port B"=1, "Port C"=2, "Ports A & B"=4, "Ports A & C"=5, "Ports B & C"=6, "All Ports"=3] ("Output Ports (A & B) 10")
            # "Attack Wheel"
            # "0 = Forward"
            n117 = call <vilib>:"SteeringOn.vi"("Power (75)"=100, "Steering (100)"=-100, "NXT/EV3"=w371, "Output Ports (A & B)"=w376) -> ("NXT/EV3"=w373:T3)
            n118 = call <vilib>:"Wait_Num(msec).vi"("Time (100 msec)"=u32 1000, "NXT/EV3"=w373) -> ()  [unwired: 2 in, 1 out]
            n119 = call <vilib>:"SteeringOn.vi"("Power (75)"=100, "Steering (100)"=0, "NXT/EV3"=w371, "Output Ports (A & B)"=w377) -> ("NXT/EV3"=w378:T3)
          }
        }
      }
    }
    n120 = Add(x=w5, y=0) -> (x+y=w3:i32)
    n121 = Not Equal To 0?(x=w3) -> (x != 0?=w2:bool)
  }
